vi "ByteArray2Int.vi"(9 "index":i32, 11 "unsigned byte array":u8[](array[numeric])) -> (3 "number":u32)   [LabVIEW 2012]
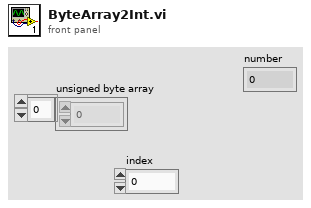
[diagram p1: front panel]
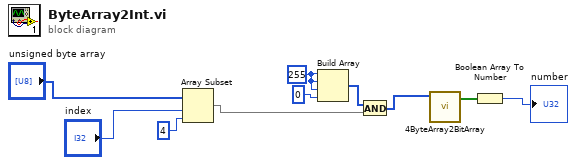
[diagram p0: block diagram]
diagram:
  w1 = u32 255 ("x*2^n")
  n1 = Array Subset(array="unsigned byte array", index="index", length=4) -> (w4:u8[])
  n2 = Build Array(w1, w1, w1, u32 0 ("x*2^n")) -> (w3:u32[])
  n3 = And(x=w3, y=w4) -> (x .and. y?=w5:u32[])
  n4 = call "4ByteArray2BitArray.vi"("array"=w5) -> ("Array"=w9:bool[])  [unwired: 10 in]
  n5 = Boolean Array To Number(Boolean array=w9) -> (number=→"number":u32)
